vi "Configure Multicarrier.vi"(6 "Stored File Name":string, 7 "Frequency Spacing (1.0000000000000E+6)":dbl=1000000.0 format="%.13e", 8 "error in (no error)":errorcluster, 9 "Carrier Number (2)":u32=2, 10 "Standard (1: NADC)":u16(ring)=1 items=["GSM"=0, "NADC"=1, "PDC"=2, "PHS"=3, "DECT"=4, "APCO 25 w/C4FM"=5, "APCO w/CQPSK"=6, "CDPD"=7, "PWT"=8, "EDGE"=9, "TETRA"=10, "Select File"=12], 11 "VISA resource name":refnum<visa-resource-name>) -> (0 "error out":errorcluster, 3 "VISA resource name out":refnum<visa-resource-name>)   [LabVIEW 2018, in "Agilent PSG MXG Series.lvlib"]
doc: "Builds a table with the specified carrier type, number of carriers and frequency spacing value, or retrieves the setup stored in the specified user file.\n\n<b>Note:</b>\nIt is applicable for N5172B/82B with <b>Option 431</b>, or N5162A, N5182A."
uses:
  Agilent PSG MXG Series.lvlib
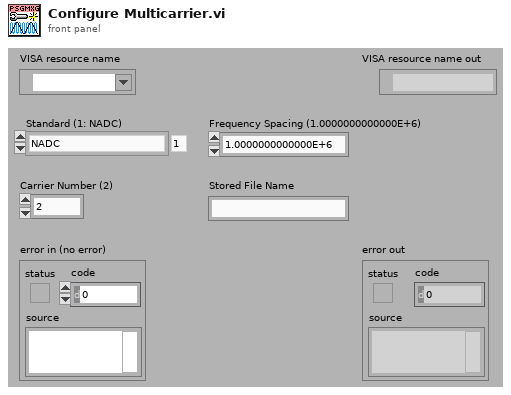
[diagram p1: front panel]
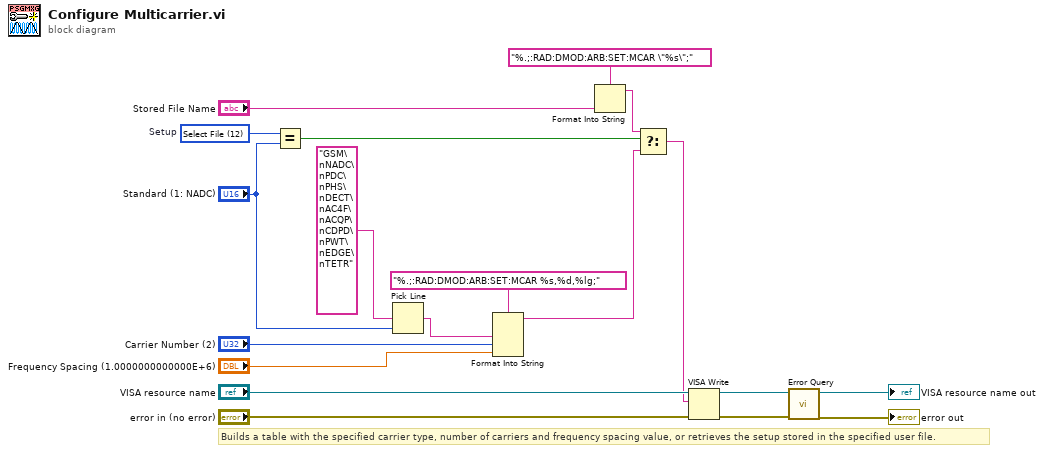
[diagram p0: block diagram]
diagram:
  w1 = u16 12 items=["GSM"=0, "NADC"=1, "PDC"=2, "PHS"=3, "DECT"=4, "APCO 25 w/C4FM"=5, "APCO w/CQPSK"=6, "CDPD"=7, "PWT"=8, "EDGE"=9, "TETRA"=10, "Select File"=12]  # Setup
  # "Builds a table with the specified carrier type, number of carriers and frequency spacing value, or retrieves the setup stored in the specified user file."
  n1 = Equal?(x=w1, y="Standard (1: NADC)") -> (x = y?=w6:bool)
  n2 = Pick Line(multi-line string="GSM\nNADC\nPDC\nPHS\nDECT\nAC4F\nACQP\nCDPD\nPWT\nEDGE\nTETR", line index="Standard (1: NADC)") -> (output string=w17:string)  [unwired: 1 in]
  n3 = Format Into String(format string="%.;:RAD:DMOD:ARB:SET:MCAR %s,%d,%lg;", w17, "Carrier Number (2)", "Frequency Spacing (1.0000000000000E+6)") -> (resulting string=w4:string)  [unwired: 2 in, 1 out]
  n4 = Format Into String(format string="%.;:RAD:DMOD:ARB:SET:MCAR \"%s\";", "Stored File Name") -> (resulting string=w5:string)  [unwired: 2 in, 1 out]
  n5 = Select(t=w5, s=w6, f=w4) -> (s? t:f=w3:string)
  n6 = VISA Write(VISA resource name="VISA resource name", write buffer=w3, error in (no error)="error in (no error)") -> (VISA resource name out=w12:refnum<visa-resource-name>, error out=w11:errorcluster)  [unwired: 1 out]
  n7 = call "Error Query.vi"("error in (no error)"=w11, "VISA resource name"=w12) -> ("error out"=→"error out":errorcluster, "VISA resource name out"=→"VISA resource name out":refnum<visa-resource-name>)  [unwired: 6 in, 2 out]
